vi "HOST_4651.vi"() -> ()   [LabVIEW 2018]
uses:
  <vilib>/userdefined/High Color/nirio_resource_hc.ctl
  <instrlib>/niDCPower/nidcpower.llb/niDCPower Measurement Type.ctl
  <vilib>/FPGAPlugInAG/PXI-7953R/niLvFpga_Open_PXI-7953R.vi
  <vilib>/rvi/interface/common/dynamic/niFpgaDynamicAddResources.vi
  <vilib>/FPGAPlugInAG/Dynamic/niLvFpga_Reset_Dynamic.vi
  <vilib>/FPGAPlugInAG/Dynamic/niLvFpga_Run_Dynamic.vi
  <vilib>/Utility/error.llb/Error Cluster From Error Code.vi
  <vilib>/rvi/errors/niLvFpgaAdjustHostInterfaceError.vi
  <vilib>/FPGAPlugInAG/Dynamic/niLvFpga_Close_Dynamic.vi
  <vilib>/rvi/interface/nirviOpenFPGA/nirviOpenFPGA.xnode
  FPGA Bitfiles/GMAX4651_FPGATarget_Target4651_7TB9TLSSPWg.lvbitx
  <vilib>/rvi/interface/nirviMethod/nirviMethod.xnode
  <vilib>/rvi/interface/nirviReadWriteControl/nirviReadWriteControl.xnode
  <vilib>/rvi/interface/nirviCloseFPGA/nirviCloseFPGA.xnode
  <vilib>/rvi/interface/Simulation/niFpgaSimulationCallBeginRW.vi
  NiFpgaLv.dll
  <vilib>/FPGAPlugInAG/Dynamic/niLvFpga_ReadFifo_Dynamic.vi
  <vilib>/rvi/errors/niLvFpgaMergeErrorWithErrorCode.vi
  <vilib>/FPGAPlugInAG/Dynamic/niLvFpga_StartFifo_Dynamic.vi
  <vilib>/FPGAPlugInAG/Dynamic/niLvFpga_WriteFifo_Dynamic.vi
panel:
  in  "Обнулить сбои":bool
  out "Прошили":bool
  out "НИ":bool
  out "FIFO_READ":i32
  out "Выкачали из памяти":bool
  in  "Проверка сбоев":bool
  out "SEU":u32
  in  "SPI":bool
  in  "Upd_WR":bool
  in  "W(T)/R(F)":bool
  out "READ":u8[](array[numeric])
  in  "Регистры":u8[](array[numeric])=[119, 12, 0, 1, 0, 0, 1, 0, 0, 0, 0, 0, 171, 23, 1, 0, 0, 4, 0, 24, 0, 120, 15, 0, 0, 0, 0, 0, 0, 0, 0, 0, 0, 0, 0, 0, 0, 0, 0, 0, 0, 0, 0, 0, 0, 0, 0, 0, 0, 0, 0, 0, 0, 0, 0, 0, 0, 0, 0, 0, 0, 0, 0, 0, 0, 0, 0, 0, 0, 0, 0, 0, 0, 0, 0, 0, 0, 0, 0, 0, 0, 0, 0, 172, 23, 0, 0, 6, 4, 4, 4, 196, 0, 32, 32, 4, 0, 5, 0, 5, 1, 4, 0, 139, 21, 255, 7, 1, 0, 0, 134, 1, 144, 2, 12, 0, 1, 236, 245, 255, 255, 114, 252, 255, 255, 255, 255, 255, 255, 255, 255, 255, 255, 255, 255, 255, 255, 255, 255, 255, 255, 118, 253, 255, 255, 255, 255, 255, 255, 255, 255, 249, 52, 244, 255, 255, 255, 255, 255, 255, 255, 255, 255, 255, 255, 255, 169, 252, 159, 202, 255, 217, 252, 159, 205, 255, 118, 253, 255, 255, 255, 118, 253, 255, 255, 255, 118, 253, 255, 255, 255, 118, 253, 255, 255, 255, 5, 196, 179, 79, 92, 5, 196, 179, 79, 92, 1, 12, 176, 192, 19, 105, 204, 245, 192, 20, 123, 220, 245, 196, 20, 115, 229, 213, 197, 255, 91, 124, 49, 192, 2, 87, 140, 241, 192, 19, 123, 220, 85, 68, 47, 5, 0, 241, 255, 255, 255, 255, 95, 192, 14, 5, 236, 0, 0, 0, 0, 0, 0, 0, 0, 0, 0, 0, 0, 0, 0, 0, 0, 0, 0, 0, 0, 0, 0, 0, 0, 0, 0, 0, 0, 0, 0, 0, 0, 0, 0, 0, 0, 0, 0, 0, 0, 0, 0, 0, 0, 0, 0, 0, 0, 0, 0, 0, 0, 0, 0, 0, 106, 1, 0, 0, 6, 27, 142, 9, 108, 57, 0, 0, 0, 0, 108, 57, 23, 15, 8, 1, 20, 0, 56, 71, 96, 68, 0, 0, 0, 0, 188, 194, 172, 160, 180, 148, 148, 200, 0, 160, 128, 148, 194, 66, 66, 64, 0, 0, 254, 254, 254, 254, 254, 254, 16, 160, 192, 0, 0, 0, 0, 0]
  in  "Адрес":u16
  in  "Кол-во":u16=370
  in  "Хватит ждать!":bool
  out "Записали адресов":u32
  out "Image":T1(plugin-control)
  out "世男":bool
  in  "FRAME!":bool
  in  "MOVIE":bool
  out "VGRSH":bool
  out "VDD33A":bool
  out "VGRSL":bool
  out "VDDCH":bool
  out "VTX1H":bool
  out "VDD33A":u16
  out "VDDCH":u16
  out "VTX1L":u16
  out "VDD13":u16
  in  "SEL_Time, ms":u32=100
  out "SEL":bool
  in  "VGRSH_selcur":dbl=0.07 caption="current limit" format="%_6p"
  in  "VDD33A_selcur":dbl=0.3 caption="current limit" format="%_6p"
  in  "VGRSL_selcur":dbl=0.03 caption="current limit" format="%_6p"
  in  "VDDCH_selcur":dbl=0.15 caption="current limit" format="%_6p"
  in  "VTX1H_selcur":dbl=0.2 caption="current limit" format="%_6p"
  in  "VTX1L_selcur":dbl=0.05 caption="current limit" format="%_6p"
  in  "VDDCL_RF_RS_selcur":dbl=0.1 caption="current limit" format="%_6p"
  in  "VDD13_selcur":dbl=0.99 caption="current limit" format="%_6p"
  in  "VDDPIX_selcur":dbl=0.5 caption="current limit" format="%_6p"
  out "VTX1L":bool
  out "VDDCL":bool
  out "VDD13":bool
  out "VDDPIX":bool
  in  "Период опроса, мс":u32=1
  in  "VDD33A, V":dbl=3.3 caption="voltage level" format="%_6p"
  in  "VDDCH, V":dbl=3.75 caption="voltage level" format="%_6p"
  in  "VTX1H, V":dbl=3.6 caption="voltage level" format="%_6p"
  in  "VDDCL_RF_RS, V":dbl=1.1 caption="voltage level" format="%_6p"
  in  "VDD33A_curlim":dbl=0.5 caption="current limit" format="%_6p"
  in  "VGRSL_curlim":dbl=0.1 caption="current limit" format="%_6p"
  in  "VDDCH_curlim":dbl=0.3 caption="current limit" format="%_6p"
  in  "VTX1H_curlim":dbl=0.3 caption="current limit" format="%_6p"
  in  "VTX1L_curlim":dbl=0.1 caption="current limit" format="%_6p"
  in  "VDDCL_RF_RS_curlim":dbl=0.2 caption="current limit" format="%_6p"
  in  "VGRSL, V":dbl=-1.0 caption="voltage level" format="%_6p"
  in  "VTX1L, V":dbl=-1.3 caption="voltage level" format="%_6p"
  out "VDD33A_char":dbl(graph)=2.9426590888639165e-06
  out "VGRSL_char":dbl(graph)=1.8968380980834295e-06
  out "VDDCH_char":dbl(graph)=0.00011100375072345994
  out "VTX1H_char":dbl(graph)=2.7759221072203326e-06
  out "VTX1L_char":dbl(graph)=-1.4343692569601055e-07
  out "VDDCL_RF_RS_char":dbl(graph)=7.705063078661294e-05
  in  "VDD13, V":dbl=1.3 caption="voltage level" format="%_6p"
  in  "VDD13_curlim":dbl=1.0 caption="current limit" format="%_6p"
  out "VDD13_char":dbl(graph)=-4.0587860431954116e-07
  in  "LED, V":dbl=-3.0 caption="voltage level" format="%_6p"
  in  "LED_curlim":dbl=0.05 caption="current limit" format="%_6p"
  out "LED_char":dbl(graph)=-1.6465603775405444e-06
  in  "VGRSH, V":dbl=4.1 caption="voltage level" format="%_6p"
  in  "VGRSH_curlim":dbl=0.1 caption="current limit" format="%_6p"
  out "VGRSH_char":dbl(graph)=7.96703589777135e-05
  in  "VDDPIX, V":dbl=3.9 caption="voltage level" format="%_6p"
  in  "VDDPIX_curlim":dbl=0.6 caption="current limit" format="%_6p"
  out "VDDPIX_char":dbl(graph)=4.6929457201886834e-05
  in  "3,3V_LVDS, V":dbl=3.3 caption="voltage level" format="%_6p"
  in  "3,3V_LVDS_curlim":dbl=0.1 caption="current limit" format="%_6p"
  out "3,3V_LVDS_char":dbl(graph)=1.0317150729546496e-06
  out "VGRSH_cur":dbl caption="measurement" format="%_6g"
  out "VDD33A_cur":dbl caption="measurement" format="%_6g"
  out "VGRSL_cur":dbl caption="measurement" format="%_6g"
  out "VDDCH_cur":dbl caption="measurement" format="%_6g"
  out "VTX1H_cur":dbl caption="measurement" format="%_6g"
  out "VTX1L_cur":dbl caption="measurement" format="%_6g"
  out "VDDCL_RF_RS_cur":dbl caption="measurement" format="%_6g"
  in  "LED":bool caption="output enabled"
  out "VDD13_cur":dbl caption="measurement" format="%_6g"
  out "VDDPIX_cur":dbl caption="measurement" format="%_6g"
  out "VGRSL":u16
  out "VDDPIX":u16
  out "VTX1H":u16
  out "VDDCL":u16
  out "VGRSH":u16
  in  "Стоп":bool
  in  "Питание":bool
  in  "SIM_SEL":bool
  in  "0":refnum<k15>="PXI1Slot2" caption="1"
  in  "1":refnum<k15>="PXI1Slot3"
  in  "2":refnum<k15>="PXI1Slot4" caption="1"
  in  "3":refnum<k15>="PXI1Slot5" caption="1"
  in  "resource name 2":T2="RIO0"
  in  "SEU":path=path "C:/LabView_PRJ/GMAX4651/SEU"
  in  "SEL":path=path "C:/LabView_PRJ/GMAX4651/SEL"
  out "Номер образца":string="0"
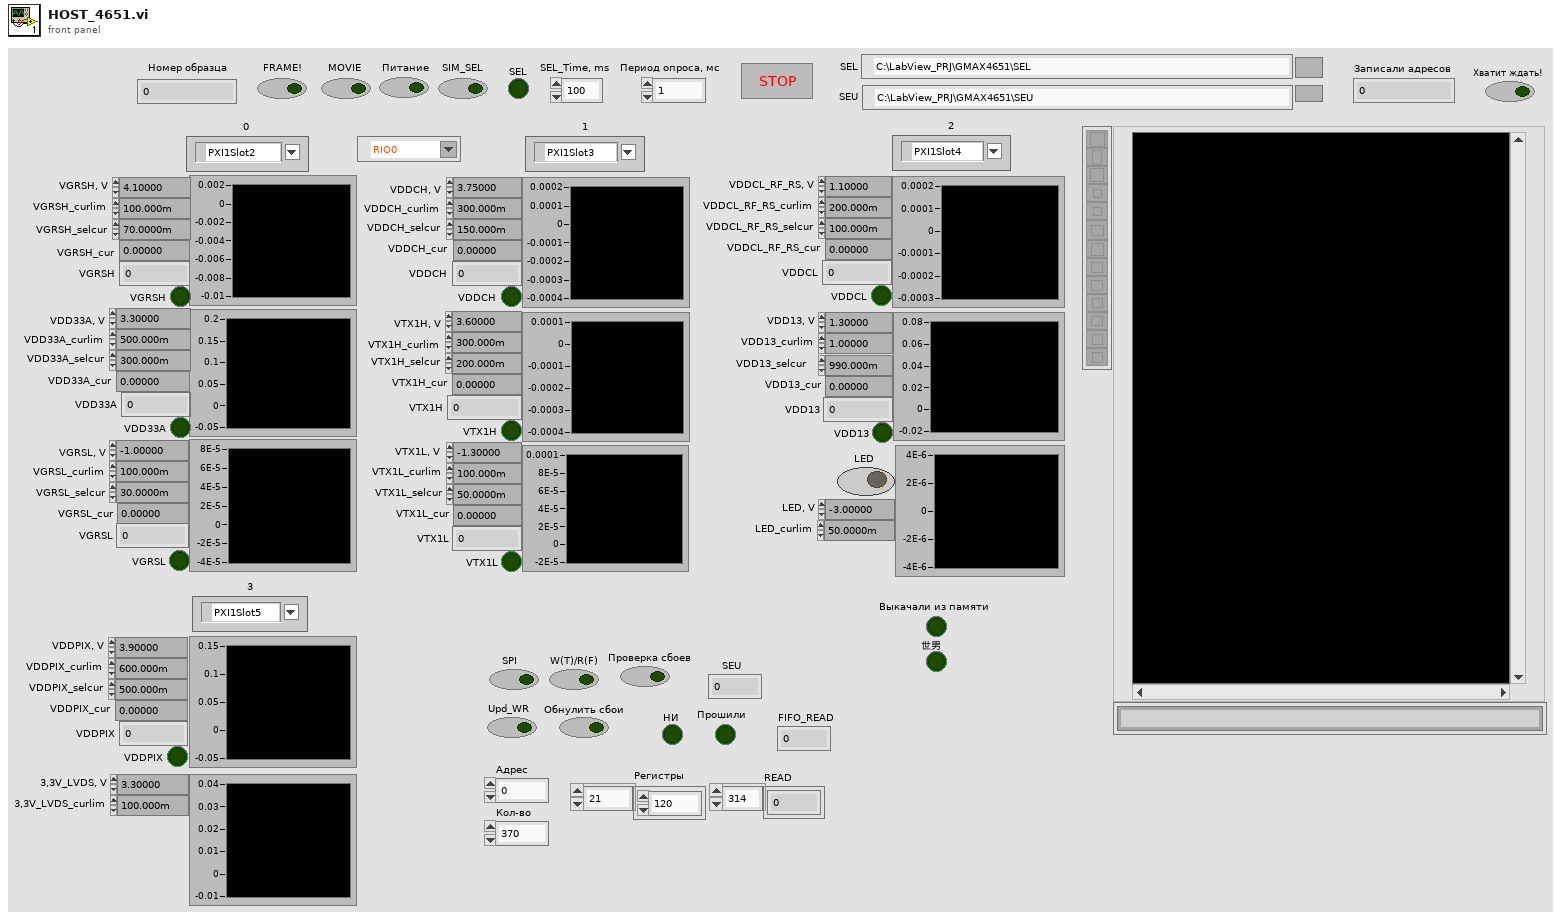
[diagram p1: front panel]
types:
  T1 = typedef "IMAQ Image.ctl" = refnum<image>
  T2 = typedef "nirio_resource_hc.ctl" = tag
  T3 = typedef "Image Type" = u32
  T4 = enum16{"open", "replace", "create", "open or create", "replace or create", "replace or create with confirmation"}
  T5 = typedef "niDCPower Measurement Type.ctl" = i32
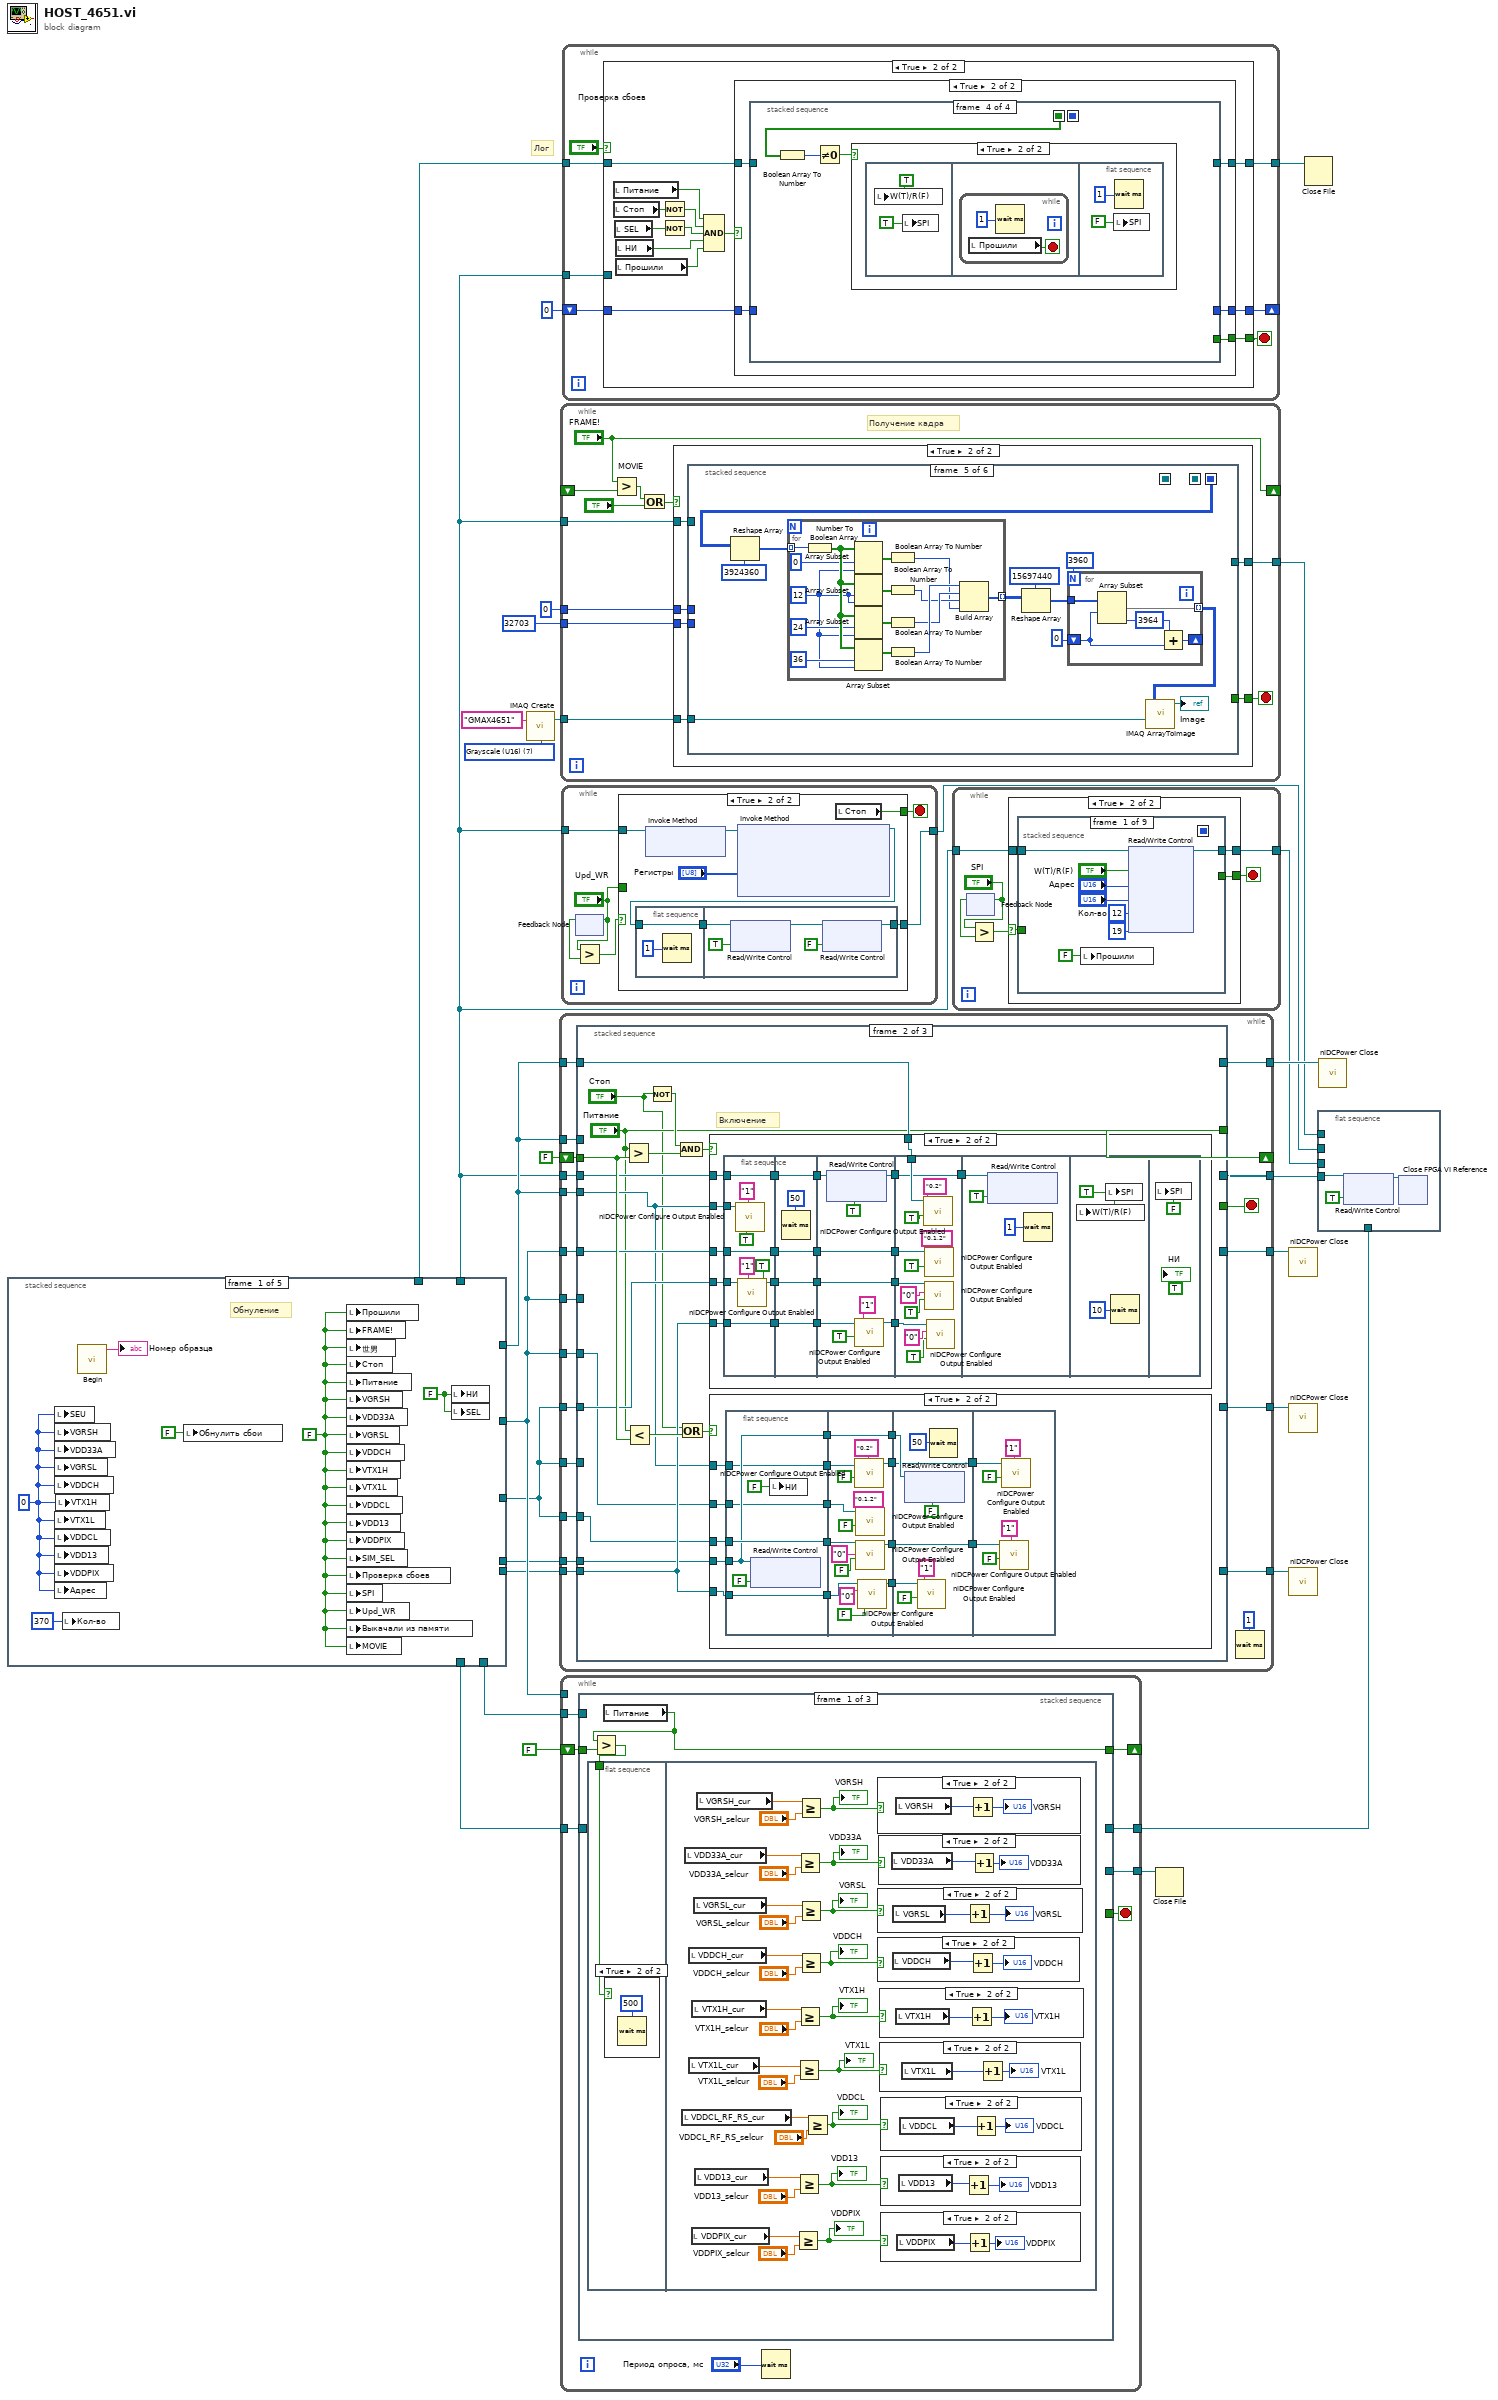
[diagram p0: block diagram]
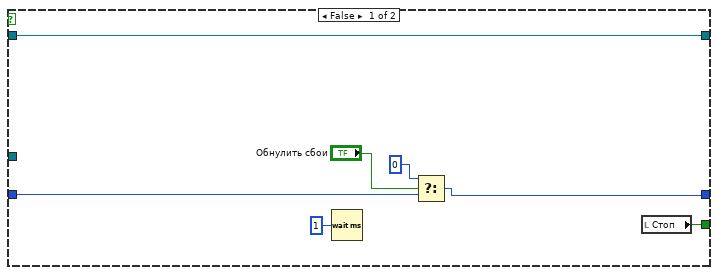
[diagram p2: hidden frame]
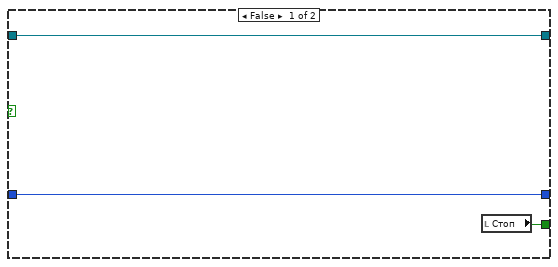
[diagram p3: hidden frame]
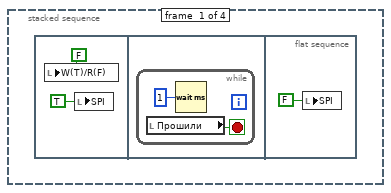
[diagram p4: hidden frame]
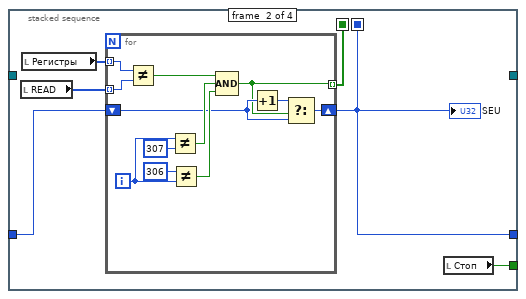
[diagram p5: hidden frame]
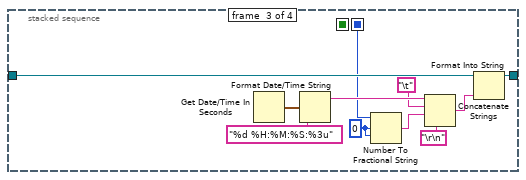
[diagram p6: hidden frame]
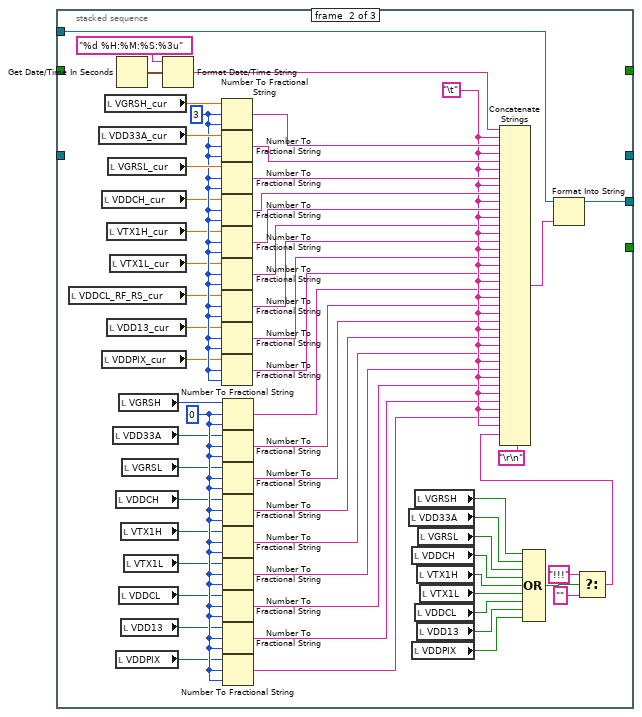
[diagram p18: hidden frame]
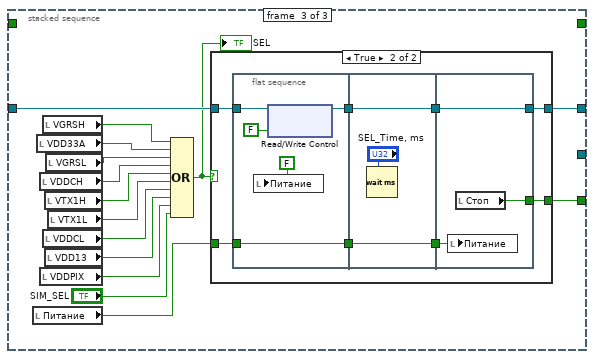
[diagram p19: hidden frame]
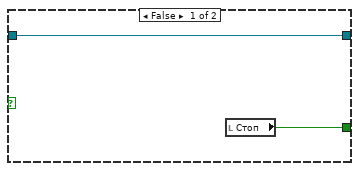
[diagram p20: hidden frame]
diagram:
  w13 = T3 7 items=["Grayscale (U8)", "Grayscale (I16)", "Grayscale (SGL)", "Complex (CSG)", "RGB (U32)", "HSL (U32)", "RGB (U64)", "Grayscale (U16)"] ("Image Type")
  # "Лог"
  n1 = stacked-sequence {
    tunnel: [_ _ _ _ w115] -> w19
    tunnel: [_ _ _ _ w108] -> w21
    tunnel: [_ _ _ _ w119] -> w20
    tunnel: [_ _ _ w103 _] -> w4
    tunnel: [_ _ _ w103 _] -> w16
    tunnel: [_ w42 _ _ _] -> w17
    tunnel: [_ _ _ _ w109] -> w18
    tunnel: [_ _ _ w103 _] -> w15
    tunnel: [_ _ w72 _ _] -> w3
    frame #0 {
      w31 = FALSE ("НИ")
      w30 = FALSE ("Стоп")
      w33 = u16 0 ("ADC")
      # "Обнуление"
      n2 = local write "SEU"(w33) -> ()
      n3 = local write "VGRSH"(w33) -> ()
      n4 = local write "VDD33A"(w33) -> ()
      n5 = local write "VGRSL"(w33) -> ()
      n6 = local write "VDDCH"(w33) -> ()
      n7 = local write "VTX1L"(w33) -> ()
      n8 = local write "VDDCL"(w33) -> ()
      n9 = local write "VDD13"(w33) -> ()
      n10 = local write "VDDPIX"(w33) -> ()
      n11 = local write "Адрес"(w33) -> ()
      n12 = local write "VTX1H"(w33) -> ()
      n13 = local write "Кол-во"(u16 370 ("Кол-во")) -> ()
      n14 = call "Begin.vi"() -> ("Номер образца 2"=→"Номер образца":string)  [unwired: 11 in]
      n15 = local write "Обнулить сбои"(FALSE ("Обнулить сбои")) -> ()
      n16 = local write "Прошили"(w30) -> ()
      n17 = local write "FRAME!"(w30) -> ()
      n18 = local write "世男"(w30) -> ()
      n19 = local write "Стоп"(w30) -> ()
      n20 = local write "Питание"(w30) -> ()
      n21 = local write "VGRSH"(w30) -> ()
      n22 = local write "VDD33A"(w30) -> ()
      n23 = local write "VGRSL"(w30) -> ()
      n24 = local write "VDDCH"(w30) -> ()
      n25 = local write "VTX1H"(w30) -> ()
      n26 = local write "VTX1L"(w30) -> ()
      n27 = local write "VDDCL"(w30) -> ()
      n28 = local write "VDD13"(w30) -> ()
      n29 = local write "VDDPIX"(w30) -> ()
      n30 = local write "SIM_SEL"(w30) -> ()
      n31 = local write "Проверка сбоев"(w30) -> ()
      n32 = local write "SPI"(w30) -> ()
      n33 = local write "Upd_WR"(w30) -> ()
      n34 = local write "Выкачали из памяти"(w30) -> ()
      n35 = local write "MOVIE"(w30) -> ()
      n36 = local write "НИ"(w31) -> ()
      n37 = local write "SEL"(w31) -> ()
    }
    frame #1 {
      w37 = "\t"
      # "Лог по токам"
      n38 = local read "Номер образца"() -> (w64:string)
      n39 = Build Path(base path="SEL", name or relative path=w64) -> (appended path=w61:path)
      n40 = Get Date/Time In Seconds() -> (seconds since 1Jan1904=w58:timestamp)
      n41 = call <vilib>:"Check if File or Folder Exists.vi"("path"=w61) -> ("file or folder exists?"=w62:bool, "dup path"=w63:path)  [unwired: 8 in, 1 out]
      n42 = Format Date/Time String(time format string (%c)="%d %H.%M.%S", seconds (now)=w58) -> (date/time string=w56:string)  [unwired: 1 in]
      n43 = case shown="False" w62 {
        tunnel: w63 -> [w70 w71]
        tunnel: [w69 w71] -> w36
        frame False {
          n44 = Create Folder(path (use dialog)=w70) -> (created path=w69:path)  [unwired: 2 in, 2 out]
        }
        frame True {
        }
      }
      n45 = Concatenate Strings(w56, ".xls" ("string")) -> (w55:string)
      n46 = Build Path(base path=w36, name or relative path=w55) -> (appended path=w57:path)
      n47 = Open/Create/Replace File(file path (use dialog)=w57, operation (0:open)=T4."open or create", access (0:read/write)=enum16{"read/write", "read-only", "write-only"}."read/write") -> (refnum out=w59:refnum<file>)  [unwired: 3 in, 2 out]
      n48 = case shown="True" TRUE {
        tunnel: w59 -> [w65 w68]
        tunnel: [w65 w66] -> w54
        frame False {
        }
        frame True {
          n49 = Set File Position(refnum=w68, from (0:start)=enum16{"start", "end", "current"}."end") -> (refnum out=w66:refnum<file>)  [unwired: 2 in, 1 out]
        }
      }
      n50 = Format Into String(initial string=w54, "Time" ("input 1"), w37, "VGRSH_cur", w37, "VDD33A_cur", w37, "VGRSL_cur", w37, "VDDCH_cur", w37, "VTX1H_cur", w37, "VTX1L_cur", w37, "VDDCL_RF_RS_cur", w37, "VDD13_cur", w37, "VDDPIX_cur", w37, "\r\n") -> (resulting string=w42:refnum<file>)  [unwired: 2 in, 1 out]
    }
    frame #2 {
      w75 = "\t"
      # "Лог по сбоям"
      n51 = local read "Номер образца"() -> (w79:string)
      n52 = Build Path(base path="SEU", name or relative path=w79) -> (appended path=w93:path)
      n53 = Get Date/Time In Seconds() -> (seconds since 1Jan1904=w91:timestamp)
      n54 = call <vilib>:"Check if File or Folder Exists.vi"("path"=w93) -> ("file or folder exists?"=w94:bool, "dup path"=w95:path)  [unwired: 8 in, 1 out]
      n55 = Format Date/Time String(time format string (%c)="%d %H.%M.%S", seconds (now)=w91) -> (date/time string=w89:string)  [unwired: 1 in]
      n56 = case shown="False" w94 {
        tunnel: w95 -> [w101 w102]
        tunnel: [w100 w102] -> w80
        frame False {
          n57 = Create Folder(path (use dialog)=w101) -> (created path=w100:path)  [unwired: 2 in, 2 out]
        }
        frame True {
        }
      }
      n58 = Concatenate Strings(w89, ".xls" ("string")) -> (w88:string)
      n59 = Build Path(base path=w80, name or relative path=w88) -> (appended path=w90:path)
      n60 = Open/Create/Replace File(file path (use dialog)=w90, operation (0:open)=T4."open or create", access (0:read/write)=enum16{"read/write", "read-only", "write-only"}."read/write") -> (refnum out=w92:refnum<file>)  [unwired: 3 in, 2 out]
      n61 = case shown="True" TRUE {
        tunnel: w92 -> [w96 w99]
        tunnel: [w96 w97] -> w87
        frame False {
        }
        frame True {
          n62 = Set File Position(refnum=w99, from (0:start)=enum16{"start", "end", "current"}."end") -> (refnum out=w97:refnum<file>)  [unwired: 2 in, 1 out]
        }
      }
      n63 = Format Into String(initial string=w87, "Time" ("input 1"), w75, "Регистр №" ("input 3"), w75, "Содержание" ("input 4"), w75, "Кол-во сбоев" ("input 7"), "\r\n") -> (resulting string=w72:refnum<file>)  [unwired: 2 in, 1 out]
    }
    frame #3 {
      n64 = xnode "Open FPGA VI Reference"("resource name"="resource name 2") -> ("FPGA VI Reference Out"=w104:refnum<k20>)  [unwired: 1 in, 1 out]
      n65 = xnode "Invoke Method"("FPGA VI Reference In"=w104) -> ("FPGA VI Reference Out"=w107:refnum<k20>, "error out"=w106:errorcluster)  [unwired: 1 in]
      n66 = xnode "Invoke Method"("FPGA VI Reference In"=w107, "error in"=w106) -> ("FPGA VI Reference Out"=w103:refnum<k20>)  [unwired: 1 in, 1 out]
    }
    frame #4 {
      n67 = call <instrlib>:"niDCPower Initialize.vi"("resource name"="2") -> ("error out"=w125:errorcluster, "instrument handle out"=w122:refnum<k15>)  [unwired: 3 in, 6 out]
      n68 = call <instrlib>:"niDCPower Initialize.vi"("resource name"="1") -> ("error out"=w123:errorcluster, "instrument handle out"=w120:refnum<k15>)  [unwired: 3 in, 6 out]
      n69 = call <instrlib>:"niDCPower Initialize.vi"("resource name"="3") -> ("error out"=w113:errorcluster, "instrument handle out"=w114:refnum<k15>)  [unwired: 3 in, 6 out]
      n70 = call <instrlib>:"niDCPower Initialize.vi"("resource name"="0") -> ("error out"=w124:errorcluster, "instrument handle out"=w121:refnum<k15>)  [unwired: 3 in, 6 out]
      n71 = call <instrlib>:"niDCPower Configure Voltage Level.vi"("error in (no error)"=w125, "voltage level"=0.0, "channel name"="0,1,2", "instrument handle"=w122) -> ("instrument handle out"=w115:refnum<k15>)  [unwired: 6 in, 1 out]
      n72 = call <instrlib>:"niDCPower Configure Voltage Level.vi"("error in (no error)"=w123, "voltage level"=0.0, "channel name"="0,1,2", "instrument handle"=w120) -> ("instrument handle out"=w119:refnum<k15>)  [unwired: 6 in, 1 out]
      n73 = call <instrlib>:"niDCPower Configure Voltage Level.vi"("error in (no error)"=w113, "voltage level"=0.0, "channel name"="0,1", "instrument handle"=w114) -> ("instrument handle out"=w109:refnum<k15>)  [unwired: 6 in, 1 out]
      n74 = call <instrlib>:"niDCPower Configure Voltage Level.vi"("error in (no error)"=w124, "voltage level"=0.0, "channel name"="0,1,2", "instrument handle"=w121) -> ("instrument handle out"=w108:refnum<k15>)  [unwired: 6 in, 1 out]
    }
  }
  n75 = call "IMAQ Create"("Image Name"="GMAX4651", "Image Type"=w13) -> ("New Image"=w10:T1)  [unwired: 3 in, 1 out]
  n76 = while {
    shift-right: [w151] -> _
    shift-left: FALSE -> [w152]
    tunnel: w21 -> [w150]
    tunnel: w20 -> [w144]
    tunnel: w19 -> [w141]
    tunnel: w18 -> [w149]
    tunnel: w21 -> [w146]
    tunnel: w21 -> [w145]
    tunnel: w20 -> [w143]
    tunnel: w20 -> [w142]
    tunnel: w19 -> [w140]
    tunnel: w19 -> [w139]
    tunnel: [w138] -> w25
    tunnel: [w137] -> w26
    tunnel: [w136] -> w27
    tunnel: [w135] -> w28
    tunnel: w4 -> [w134]
    tunnel: w15 -> [w133]
    tunnel: [w132] -> w5
    stop <- w148 stop-if-true
    n77 = stacked-sequence {
      tunnel: w152 -> [_ w271 _]
      tunnel: [_ "Питание" _] -> w151
      tunnel: w150 -> [w164 w258 w392]
      tunnel: w149 -> [w153 w263 w389]
      tunnel: [_ _ w393] -> w148
      tunnel: w146 -> [w163 _ _]
      tunnel: w145 -> [w162 w260 _]
      tunnel: w144 -> [w161 w266 w391]
      tunnel: w143 -> [w160 _ _]
      tunnel: w142 -> [w159 w261 _]
      tunnel: w141 -> [w158 w265 w390]
      tunnel: w140 -> [w157 _ _]
      tunnel: w139 -> [w156 w262 _]
      tunnel: [_ _ w392] -> w138
      tunnel: [_ _ w391] -> w137
      tunnel: [_ _ w390] -> w136
      tunnel: [_ _ w389] -> w135
      tunnel: w134 -> [_ w259 w388]
      tunnel: w133 -> [_ w257 _]
      tunnel: [_ _ w388] -> w132
      frame #0 {
        w178 = T5 0 items=["Current", "Voltage"] ("measurement type")
        n78 = call <instrlib>:"niDCPower Configure Current Limit.vi"("current limit"="VGRSH_curlim", "channel name"="0", "instrument handle"=w164) -> ("instrument handle out"=w195:refnum<k15>)  [unwired: 7 in, 1 out]
        n79 = call <instrlib>:"niDCPower Configure Current Limit.vi"("current limit"="VDD33A_curlim", "channel name"="1", "instrument handle"=w163) -> ("instrument handle out"=w235:refnum<k15>)  [unwired: 7 in, 1 out]
        n80 = call <instrlib>:"niDCPower Configure Current Limit.vi"("current limit"="VGRSL_curlim", "channel name"="2", "instrument handle"=w162) -> ("instrument handle out"=w236:refnum<k15>)  [unwired: 7 in, 1 out]
        n81 = call <instrlib>:"niDCPower Configure Current Limit.vi"("current limit"="VDDCH_curlim", "channel name"="0", "instrument handle"=w161) -> ("instrument handle out"=w237:refnum<k15>)  [unwired: 7 in, 1 out]
        n82 = call <instrlib>:"niDCPower Configure Current Limit.vi"("current limit"="VTX1H_curlim", "channel name"="1", "instrument handle"=w160) -> ("instrument handle out"=w238:refnum<k15>)  [unwired: 7 in, 1 out]
        n83 = call <instrlib>:"niDCPower Configure Current Limit.vi"("current limit"="VTX1L_curlim", "channel name"="2", "instrument handle"=w159) -> ("instrument handle out"=w239:refnum<k15>)  [unwired: 7 in, 1 out]
        n84 = call <instrlib>:"niDCPower Configure Current Limit.vi"("current limit"="VDDCL_RF_RS_curlim", "channel name"="0", "instrument handle"=w158) -> ("instrument handle out"=w240:refnum<k15>)  [unwired: 7 in, 1 out]
        n85 = call <instrlib>:"niDCPower Configure Current Limit.vi"("current limit"="VDD13_curlim", "channel name"="1", "instrument handle"=w157) -> ("instrument handle out"=w208:refnum<k15>)  [unwired: 7 in, 1 out]
        n86 = call <instrlib>:"niDCPower Configure Current Limit.vi"("current limit"="LED_curlim", "channel name"="2", "instrument handle"=w156) -> ("instrument handle out"=w203:refnum<k15>)  [unwired: 7 in, 1 out]
        n87 = call <instrlib>:"niDCPower Configure Current Limit.vi"("current limit"="VDDPIX_curlim", "channel name"="0", "instrument handle"=w153) -> ("instrument handle out"=w188:refnum<k15>)  [unwired: 7 in, 1 out]
        n88 = call <instrlib>:"niDCPower Configure Current Limit.vi"("current limit"="3,3V_LVDS_curlim", "channel name"="1", "instrument handle"=w153) -> ("instrument handle out"=w183:refnum<k15>)  [unwired: 7 in, 1 out]
        n89 = call <instrlib>:"niDCPower Configure Voltage Level.vi"("voltage level"="VGRSH, V", "channel name"="0", "instrument handle"=w195) -> ("instrument handle out"=w198:refnum<k15>)  [unwired: 7 in, 1 out]
        n90 = call <instrlib>:"niDCPower Configure Voltage Level.vi"("voltage level"="VDD33A, V", "channel name"="1", "instrument handle"=w235) -> ("instrument handle out"=w218:refnum<k15>)  [unwired: 7 in, 1 out]
        n91 = call <instrlib>:"niDCPower Configure Voltage Level.vi"("voltage level"="VGRSL, V", "channel name"="2", "instrument handle"=w236) -> ("instrument handle out"=w217:refnum<k15>)  [unwired: 7 in, 1 out]
        n92 = call <instrlib>:"niDCPower Configure Voltage Level.vi"("voltage level"="VDDCH, V", "channel name"="0", "instrument handle"=w237) -> ("instrument handle out"=w216:refnum<k15>)  [unwired: 7 in, 1 out]
        n93 = call <instrlib>:"niDCPower Configure Voltage Level.vi"("voltage level"="VTX1H, V", "channel name"="1", "instrument handle"=w238) -> ("instrument handle out"=w215:refnum<k15>)  [unwired: 7 in, 1 out]
        n94 = call <instrlib>:"niDCPower Configure Voltage Level.vi"("voltage level"="VTX1L, V", "channel name"="2", "instrument handle"=w239) -> ("instrument handle out"=w214:refnum<k15>)  [unwired: 7 in, 1 out]
        n95 = call <instrlib>:"niDCPower Configure Voltage Level.vi"("voltage level"="VDDCL_RF_RS, V", "channel name"="0", "instrument handle"=w240) -> ("instrument handle out"=w213:refnum<k15>)  [unwired: 7 in, 1 out]
        n96 = call <instrlib>:"niDCPower Configure Voltage Level.vi"("voltage level"="VDD13, V", "channel name"="1", "instrument handle"=w208) -> ("instrument handle out"=w211:refnum<k15>)  [unwired: 7 in, 1 out]
        n97 = call <instrlib>:"niDCPower Configure Voltage Level.vi"("voltage level"="LED, V", "channel name"="2", "instrument handle"=w203) -> ("instrument handle out"=w200:refnum<k15>)  [unwired: 7 in, 1 out]
        n98 = call <instrlib>:"niDCPower Configure Voltage Level.vi"("voltage level"="VDDPIX, V", "channel name"="0", "instrument handle"=w188) -> ("instrument handle out"=w191:refnum<k15>)  [unwired: 7 in, 1 out]
        n99 = call <instrlib>:"niDCPower Configure Voltage Level.vi"("voltage level"="3,3V_LVDS, V", "channel name"="1", "instrument handle"=w183) -> ("instrument handle out"=w180:refnum<k15>)  [unwired: 7 in, 1 out]
        n100 = call <instrlib>:"niDCPower Measure.vi"("measurement type"=w178, "channel name"="0", "instrument handle"=w198) -> ("measurement"=→"VGRSH_char" →"VGRSH_cur":dbl)  [unwired: 6 in, 2 out]
        n101 = call <instrlib>:"niDCPower Measure.vi"("measurement type"=w178, "channel name"="1", "instrument handle"=w218) -> ("measurement"=→"VDD33A_char" →"VDD33A_cur":dbl)  [unwired: 6 in, 2 out]
        n102 = call <instrlib>:"niDCPower Measure.vi"("measurement type"=w178, "channel name"="2", "instrument handle"=w217) -> ("measurement"=→"VGRSL_char" →"VGRSL_cur":dbl)  [unwired: 6 in, 2 out]
        n103 = call <instrlib>:"niDCPower Measure.vi"("measurement type"=w178, "channel name"="0", "instrument handle"=w216) -> ("measurement"=→"VDDCH_char" →"VDDCH_cur":dbl)  [unwired: 6 in, 2 out]
        n104 = call <instrlib>:"niDCPower Measure.vi"("measurement type"=w178, "channel name"="1", "instrument handle"=w215) -> ("measurement"=→"VTX1H_char" →"VTX1H_cur":dbl)  [unwired: 6 in, 2 out]
        n105 = call <instrlib>:"niDCPower Measure.vi"("measurement type"=w178, "channel name"="2", "instrument handle"=w214) -> ("measurement"=→"VTX1L_char" →"VTX1L_cur":dbl)  [unwired: 6 in, 2 out]
        n106 = call <instrlib>:"niDCPower Measure.vi"("measurement type"=w178, "channel name"="0", "instrument handle"=w213) -> ("measurement"=→"VDDCL_RF_RS_char" →"VDDCL_RF_RS_cur":dbl)  [unwired: 6 in, 2 out]
        n107 = call <instrlib>:"niDCPower Measure.vi"("measurement type"=w178, "channel name"="1", "instrument handle"=w211) -> ("measurement"=→"VDD13_char" →"VDD13_cur":dbl)  [unwired: 6 in, 2 out]
        n108 = call <instrlib>:"niDCPower Measure.vi"("measurement type"=w178, "channel name"="2", "instrument handle"=w200) -> ("measurement"=→"LED_char":dbl, "instrument handle out"=w166:refnum<k15>)  [unwired: 6 in, 1 out]
        n109 = call <instrlib>:"niDCPower Measure.vi"("measurement type"=w178, "channel name"="0", "instrument handle"=w191) -> ("measurement"=→"VDDPIX_char" →"VDDPIX_cur":dbl)  [unwired: 6 in, 2 out]
        n110 = call <instrlib>:"niDCPower Measure.vi"("measurement type"=w178, "channel name"="1", "instrument handle"=w180) -> ("measurement"=→"3,3V_LVDS_char":dbl)  [unwired: 6 in, 2 out]
        n111 = call <instrlib>:"niDCPower Configure Output Enabled.vi"("output enabled"="LED", "channel name"="2", "instrument handle"=w166) -> ()  [unwired: 7 in, 2 out]
      }
      frame #1 {
        # "Включение"
        n112 = Greater?(x="Питание", y=w271) -> (0:w269:bool)
        n113 = Less?(x="Питание", y=w271) -> (x < y?=w267:bool)
        n114 = Not(x="Стоп") -> (.not. x?=w268:bool)
        n115 = And(x=w268, y=w269) -> (x .and. y?=w270:bool)
        n116 = Or(x="Стоп", y=w267) -> (x .or. y?=w264:bool)
        n117 = case shown="True" w270 {
          tunnel: w266 -> [_ w336]
          tunnel: w265 -> [_ w342]
          tunnel: w260 -> [_ w343]
          tunnel: w263 -> [_ w330]
          tunnel: w259 -> [_ w341]
          tunnel: w258 -> [_ w338]
          frame False {
          }
          frame True {
            n118 = flat-sequence {
              tunnel: w343 -> [w353]
              tunnel: w342 -> [w350]
              tunnel: w341 -> [w347]
              tunnel: [w347] -> w339
              tunnel: [w346] -> w337
              tunnel: w336 -> [w346]
              tunnel: [w345] -> w331
              tunnel: w330 -> [w344]
              tunnel: [w344] -> w329
              tunnel: [w357] -> w340
              tunnel: w339 -> [w357]
              tunnel: w337 -> [w356]
              tunnel: [w356] -> w335
              tunnel: [w355] -> w332
              tunnel: w331 -> [w355]
              tunnel: w329 -> [w354]
              tunnel: [w354] -> w328
              tunnel: w340 -> [w367]
              tunnel: w335 -> [w365]
              tunnel: [w365] -> w334
              tunnel: [w364] -> w333
              tunnel: w332 -> [w364]
              tunnel: w328 -> [w362]
              tunnel: [w361] -> w327
              tunnel: [w363] -> w325
              tunnel: w338 -> [w379]
              tunnel: w334 -> [w377]
              tunnel: w333 -> [w372]
              tunnel: w327 -> [w370]
              tunnel: [w368] -> w326
              tunnel: w325 -> [w368]
              tunnel: w326 -> [w383]
              frame #0 {
                n119 = call <instrlib>:"niDCPower Configure Output Enabled.vi"("output enabled"=TRUE, "channel name"="1", "instrument handle"=w353) -> ()  [unwired: 7 in, 2 out]
                n120 = call <instrlib>:"niDCPower Configure Output Enabled.vi"("output enabled"=TRUE, "channel name"="1", "instrument handle"=w350) -> ("instrument handle out"=w345:refnum<k15>)  [unwired: 7 in, 1 out]
              }
              frame #1 {
                n121 = Wait (ms)(milliseconds to wait=u32 50) -> ()  [unwired: 1 out]
              }
              frame #2 {
                n122 = xnode "Read/Write Control"("FPGA VI Reference In"=w367, "Автомат"=TRUE) -> ("FPGA VI Reference Out"=w363:refnum<k20>)  [unwired: 1 in, 1 out]
                n123 = call <instrlib>:"niDCPower Configure Output Enabled.vi"("output enabled"=TRUE, "channel name"="1", "instrument handle"=w362) -> ("instrument handle out"=w361:refnum<k15>)  [unwired: 7 in, 1 out]
              }
              frame #3 {
                n124 = call <instrlib>:"niDCPower Configure Output Enabled.vi"("output enabled"=TRUE, "channel name"="0,2", "instrument handle"=w379) -> ()  [unwired: 7 in, 2 out]
                n125 = call <instrlib>:"niDCPower Configure Output Enabled.vi"("output enabled"=TRUE, "channel name"="0,1,2", "instrument handle"=w377) -> ()  [unwired: 7 in, 2 out]
                n126 = call <instrlib>:"niDCPower Configure Output Enabled.vi"("output enabled"=TRUE, "channel name"="0", "instrument handle"=w372) -> ()  [unwired: 7 in, 2 out]
                n127 = call <instrlib>:"niDCPower Configure Output Enabled.vi"("output enabled"=TRUE, "channel name"="0", "instrument handle"=w370) -> ()  [unwired: 7 in, 2 out]
              }
              frame #4 {
                n128 = xnode "Read/Write Control"("FPGA VI Reference In"=w383, "SYS_RST_N"=TRUE) -> ()  [unwired: 1 in, 2 out]
                n129 = Wait (ms)(milliseconds to wait=u32 1) -> ()  [unwired: 1 out]
              }
              frame #5 {
                w384 = TRUE ("SPI")
                n130 = local write "W(T)/R(F)"(w384) -> ()
                n131 = local write "SPI"(w384) -> ()
                n132 = Wait (ms)(milliseconds to wait=u32 10) -> ()  [unwired: 1 out]
              }
              frame #6 {
                n133 = local write "SPI"(FALSE ("SPI")) -> ()
                "НИ" <- TRUE ("НИ")
              }
            }
          }
        }
        n134 = case shown="True" w264 {
          tunnel: w261 -> [_ w277]
          tunnel: w262 -> [_ w283]
          tunnel: w260 -> [_ w279]
          tunnel: w263 -> [_ w285]
          tunnel: w257 -> [_ w287]
          frame False {
          }
          frame True {
            n135 = flat-sequence {
              tunnel: w287 -> [w291]
              tunnel: [w293] -> w286
              tunnel: w285 -> [w293]
              tunnel: [w292] -> w284
              tunnel: w283 -> [w292]
              tunnel: [w291] -> w281
              tunnel: [w290] -> w280
              tunnel: w279 -> [w290]
              tunnel: [w289] -> w278
              tunnel: w277 -> [w289]
              tunnel: w286 -> [w304]
              tunnel: w284 -> [w303]
              tunnel: [w302] -> w282
              tunnel: w281 -> [w302]
              tunnel: w280 -> [w301]
              tunnel: w278 -> [w300]
              tunnel: [w297] -> w275
              tunnel: [w296] -> w273
              tunnel: [w295] -> w272
              tunnel: w282 -> [w317]
              tunnel: [w315] -> w276
              tunnel: w275 -> [w315]
              tunnel: [w314] -> w274
              tunnel: w273 -> [w314]
              tunnel: w272 -> [w313]
              tunnel: w276 -> [w322]
              tunnel: w274 -> [w321]
              frame #0 {
                n136 = xnode "Read/Write Control"("FPGA VI Reference In"=w291, "SYS_RST_N"=FALSE) -> ()  [unwired: 1 in, 2 out]
                n137 = local write "НИ"(FALSE ("НИ")) -> ()
              }
              frame #1 {
                n138 = call <instrlib>:"niDCPower Configure Output Enabled.vi"("output enabled"=FALSE, "channel name"="0,2", "instrument handle"=w301) -> ("instrument handle out"=w297:refnum<k15>)  [unwired: 7 in, 1 out]
                n139 = call <instrlib>:"niDCPower Configure Output Enabled.vi"("output enabled"=FALSE, "channel name"="0,1,2", "instrument handle"=w300) -> ()  [unwired: 7 in, 2 out]
                n140 = call <instrlib>:"niDCPower Configure Output Enabled.vi"("output enabled"=FALSE, "channel name"="0", "instrument handle"=w303) -> ("instrument handle out"=w296:refnum<k15>)  [unwired: 7 in, 1 out]
                n141 = call <instrlib>:"niDCPower Configure Output Enabled.vi"("output enabled"=FALSE, "channel name"="0", "instrument handle"=w304) -> ("instrument handle out"=w295:refnum<k15>)  [unwired: 7 in, 1 out]
              }
              frame #2 {
                n142 = xnode "Read/Write Control"("FPGA VI Reference In"=w317, "Автомат"=FALSE) -> ()  [unwired: 1 in, 2 out]
                n143 = call <instrlib>:"niDCPower Configure Output Enabled.vi"("output enabled"=FALSE, "channel name"="1", "instrument handle"=w313) -> ()  [unwired: 7 in, 2 out]
                n144 = Wait (ms)(milliseconds to wait=u32 50) -> ()  [unwired: 1 out]
              }
              frame #3 {
                n145 = call <instrlib>:"niDCPower Configure Output Enabled.vi"("output enabled"=FALSE, "channel name"="1", "instrument handle"=w321) -> ()  [unwired: 7 in, 2 out]
                n146 = call <instrlib>:"niDCPower Configure Output Enabled.vi"("output enabled"=FALSE, "channel name"="1", "instrument handle"=w322) -> ()  [unwired: 7 in, 2 out]
              }
            }
          }
        }
      }
      frame #2 {
        n147 = local read "Стоп"() -> (w393:bool)
      }
    }
    n148 = Wait (ms)(milliseconds to wait=u32 1) -> ()  [unwired: 1 out]
  }
  n149 = while {
    tunnel: w4 -> [w395]
    shift-right: ["FRAME!"] -> _
    shift-left: _ -> [w404]
    tunnel: u32 0 -> [w401]
    tunnel: u32 32703 ("163840") -> [w400]
    tunnel: w10 -> [w397]
    tunnel: [w394] -> w6
    stop <- w396 stop-if-true
    # "Получение кадра"
    n150 = Greater?(x="FRAME!", y=w404) -> (0:w403:bool)
    n151 = Or(x=w403, y="MOVIE") -> (x .or. y?=w402:bool)
    n152 = case shown="True" w402 {
      tunnel: w401 -> [_ w413]
      tunnel: w400 -> [_ w412]
      tunnel: w397 -> [_ w411]
      tunnel: [w406 w410] -> w396
      tunnel: w395 -> [w405 w409]
      tunnel: [w405 w408] -> w394
      frame False {
        n153 = Wait (ms)(milliseconds to wait=u32 1) -> ()  [unwired: 1 out]
        n154 = local read "Стоп"() -> (w406:bool)
      }
      frame True {
        n155 = stacked-sequence {
          seq-local: [w416 _ _ _ _ _] -> [_ w434 _ _ _ _]
          seq-local: [_ w433 _ _ _ _] -> [_ _ w446 _ _ _]
          seq-local: [_ _ w444 _ _ _] -> [_ _ _ _ w500 _]
          tunnel: w413 -> [_ _ w447 _ _ _]
          tunnel: w412 -> [_ _ w445 _ _ _]
          tunnel: w411 -> [_ _ _ _ w492 _]
          tunnel: [_ _ _ _ _ w523] -> w410
          tunnel: w409 -> [w414 _ _ _ _ _]
          tunnel: [_ _ w443 _ _ _] -> w408
          frame #0 {
            # "Почистили FIFO"
            n156 = xnode "Invoke Method"("FPGA VI Reference In"=w414, "Number of Elements"=u32 0, "Timeout (ms)"=0) -> ("FPGA VI Reference Out"=w418:refnum<k20>, "Elements Remaining"=w419:u32)  [unwired: 1 in, 2 out]
            n157 = xnode "Invoke Method"("FPGA VI Reference In"=w418, "Number of Elements"=w419, "Timeout (ms)"=0) -> ("FPGA VI Reference Out"=w417:refnum<k20>)  [unwired: 1 in, 3 out]
            n158 = flat-sequence {
              tunnel: w417 -> [w428]
              tunnel: [w424] -> w415
              tunnel: [w430] -> w416
              tunnel: w415 -> [w429]
              frame #0 {
                n159 = xnode "Read/Write Control"("FPGA VI Reference In"=w428, "Кадр в память"=TRUE ("EXPOSURE")) -> ("FPGA VI Reference Out"=w424:refnum<k20>)  [unwired: 1 in, 1 out]
                n160 = Wait (ms)(milliseconds to wait=u32 1) -> ()  [unwired: 1 out]
                "世男" <- FALSE
                "Выкачали из памяти" <- FALSE ("Выкачали из памяти")
              }
              frame #1 {
                n161 = xnode "Read/Write Control"("FPGA VI Reference In"=w429, "Кадр в память"=FALSE) -> ("FPGA VI Reference Out"=w430:refnum<k20>)  [unwired: 1 in, 1 out]
                n162 = Wait (ms)(milliseconds to wait=u32 1) -> ()  [unwired: 1 out]
              }
            }
          }
          frame #1 {
            n163 = while {
              tunnel: [w441] -> w433
              tunnel: w434 -> [w440]
              stop <- w437 stop-if-true
              n164 = xnode "Read/Write Control"("FPGA VI Reference In"=w440) -> ("FPGA VI Reference Out"=w441:refnum<k20>, "Записали адресов"=w436:u32)  [unwired: 1 in, 1 out]
              "Записали адресов" <- w436
              n165 = Wait (ms)(milliseconds to wait=u32 1) -> ()  [unwired: 1 out]
              n166 = Greater?(x=w436, y=u32 3924000) -> (0:w438:bool)
              n167 = Or(x=w438, y="Хватит ждать!") -> (x .or. y?=w437:bool)
            }
          }
          frame #2 {
            n168 = for {
              N: 120 -> [_]
              tunnel: w446 -> [w456]
              shift-right: [w453] -> _
              shift-left: w447 -> [w455]
              shift-right: [w452] -> _
              shift-left: w445 -> [w454]
              tunnel: [w451] -> w444 mode=indexing
              tunnel: [w450] -> w443
              tunnel: w445 -> [w449]
              n169 = stacked-sequence {
                seq-local: [w458 _ _ _ _] -> [_ w465 _ _ _]
                seq-local: [_ w464 _ _ _] -> [_ _ w468 _ _]
                seq-local: [_ _ w467 _ _] -> [_ _ _ w472 _]
                seq-local: [_ _ _ w471 _] -> [_ _ _ _ w483]
                tunnel: w456 -> [w463 _ _ _ _]
                tunnel: w455 -> [w462 _ _ _ _]
                tunnel: w454 -> [w461 _ _ _ _]
                tunnel: [w460 _ _ _ _] -> w453
                tunnel: [w459 _ _ _ _] -> w452
                tunnel: [_ _ _ _ w485] -> w451
                tunnel: [_ _ _ _ w484] -> w450
                tunnel: w449 -> [w457 _ _ _ _]
                frame #0 {
                  n170 = xnode "Read/Write Control"("FPGA VI Reference In"=w463, "Нач_адр"=w462, "Кон_адр"=w461) -> ("FPGA VI Reference Out"=w458:refnum<k20>)  [unwired: 1 in, 1 out]
                  n171 = Add(x=w462, y=w457) -> (x+y=w460:u32)
                  n172 = Add(x=w457, y=w461) -> (x+y=w459:u32)
                }
                frame #1 {
                  n173 = xnode "Read/Write Control"("FPGA VI Reference In"=w465, "Кадр на ПК"=TRUE ("HOST")) -> ("FPGA VI Reference Out"=w464:refnum<k20>)  [unwired: 1 in, 1 out]
                }
                frame #2 {
                  n174 = xnode "Read/Write Control"("FPGA VI Reference In"=w468, "Кадр на ПК"=FALSE ("HOST")) -> ("FPGA VI Reference Out"=w467:refnum<k20>)  [unwired: 1 in, 1 out]
                }
                frame #3 {
                  n175 = Get Date/Time In Seconds() -> (seconds since 1Jan1904=w470:timestamp)
                  n176 = while {
                    tunnel: w472 -> [w481]
                    tunnel: [w480] -> w471
                    tunnel: w470 -> [w478]
                    stop <- w473 stop-if-true
                    # "Записан FIFO?"
                    n177 = Get Date/Time In Seconds() -> (seconds since 1Jan1904=w479:timestamp)
                    n178 = xnode "Read/Write Control"("FPGA VI Reference In"=w481) -> ("FPGA VI Reference Out"=w480:refnum<k20>, "Записали FIFO"=w475:bool)  [unwired: 1 in, 1 out]
                    n179 = Subtract(x=w479, y=w478) -> (x-y=w477:dbl)
                    n180 = Greater?(x=w477, y=5.0) -> (0:w474:bool)
                    n181 = Or(x=w475, y=w474) -> (x .or. y?=w473:bool)
                    n182 = Wait (ms)(milliseconds to wait=u32 1) -> ()  [unwired: 1 out]
                  }
                }
                frame #4 {
                  n183 = xnode "Invoke Method"("FPGA VI Reference In"=w483, "Number of Elements"=u32 0, "Timeout (ms)"=0) -> ("FPGA VI Reference Out"=w489:refnum<k20>, "Elements Remaining"=w490:u32)  [unwired: 1 in, 2 out]
                  n184 = xnode "Invoke Method"("FPGA VI Reference In"=w489, "Number of Elements"=w490, "Timeout (ms)"=0) -> ("FPGA VI Reference Out"=w484:refnum<k20>, "Data"=w485:u64[])  [unwired: 1 in, 2 out]
                }
              }
            }
          }
          frame #3 {
            n185 = local write "Выкачали из памяти"(TRUE ("Выкачали из памяти")) -> ()
          }
          frame #4 {
            n186 = Reshape Array(w500, 3924360 ("dimension size")) -> (w502:u64[])
            n187 = for {
              tunnel: w502 -> [w522] mode=indexing
              tunnel: [w516] -> w499 mode=indexing
              w517 = 12 ("index")
              n188 = Number To Boolean Array(number=w522) -> (Boolean array=w521:bool[])
              n189 = Array Subset(array=w521, index=0, length=w517) -> (w511:bool[])
              n190 = Array Subset(array=w521, index=w517, length=w517) -> (w510:bool[])
              n191 = Array Subset(array=w521, index=24, length=w517) -> (w509:bool[])
              n192 = Array Subset(array=w521, index=36, length=w517) -> (w508:bool[])
              n193 = Boolean Array To Number(Boolean array=w511) -> (number=w512:u16)
              n194 = Boolean Array To Number(Boolean array=w510) -> (number=w513:u16)
              n195 = Boolean Array To Number(Boolean array=w509) -> (number=w514:u16)
              n196 = Boolean Array To Number(Boolean array=w508) -> (number=w515:u16)
              n197 = Build Array(w515, w514, w513, w512) -> (w516:u16[])
            }
            n198 = Reshape Array(w499, 15697440 ("dimension size")) -> (w493:u16[])
            n199 = for {
              N: 3960 ("6032") -> [_]
              shift-right: [w507] -> _
              shift-left: 0 ("index") -> [w506]
              tunnel: [w505] -> w497 mode=indexing
              tunnel: w493 -> [w503]
              w504 = 3964 ("3964")
              n200 = Array Subset(array=w503, index=w506, length=w504) -> (w505:u16[])
              n201 = Add(x=w504, y=w506) -> (x+y=w507:i32)
            }
            n202 = call "IMAQ ArrayToImage"("Image Pixels (U16)"=w497, "Image"=w492) -> ("Image Out"=→"Image":T1)  [unwired: 8 in, 1 out]
          }
          frame #5 {
            n203 = local write "世男"(TRUE ("世男")) -> ()
            n204 = local read "Стоп"() -> (w523:bool)
          }
        }
      }
    }
  }
  n205 = while {
    tunnel: w16 -> [w527]
    shift-right: [w531] -> _
    shift-left: FALSE ("Питание") -> [w532]
    tunnel: w17 -> [w529]
    tunnel: [w526] -> w23
    tunnel: [w525] -> w9
    tunnel: w20 -> [_]
    stop <- w528 stop-if-true
    n206 = stacked-sequence {
      tunnel: w532 -> [w535 _ _]
      tunnel: [w534 _ _] -> w531
      tunnel: w529 -> [_ w636 _]
      tunnel: [_ _ w656] -> w528
      tunnel: w527 -> [_ _ w655]
      tunnel: [_ w625 _] -> w526
      tunnel: [_ _ w653] -> w525
      frame #0 {
        n207 = flat-sequence {
          tunnel: w533 -> [w536]
          frame #0 {
            n208 = case shown="True" w536 {
              frame False {
              }
              frame True {
                n209 = Wait (ms)(milliseconds to wait=u32 500) -> ()  [unwired: 1 out]
              }
            }
          }
          frame #1 {
            n210 = local read "VDDCL_RF_RS_cur"() -> (w549:dbl)
            n211 = local read "VDD33A_cur"() -> (w558:dbl)
            n212 = local read "VDDCH_cur"() -> (w560:dbl)
            n213 = local read "VTX1L_cur"() -> (w550:dbl)
            n214 = local read "VDDPIX_cur"() -> (w547:dbl)
            n215 = local read "VTX1H_cur"() -> (w551:dbl)
            n216 = local read "VGRSL_cur"() -> (w559:dbl)
            n217 = local read "VDD13_cur"() -> (w548:dbl)
            n218 = local read "VGRSH_cur"() -> (w557:dbl)
            n219 = Greater Or Equal?(x=w547, y="VDDPIX_selcur") -> (x >= y?=w543:bool)
            "VDDPIX" <- w543
            n220 = Greater Or Equal?(x=w550, y="VTX1L_selcur") -> (x >= y?=w546:bool)
            "VTX1L" <- w546
            n221 = Greater Or Equal?(x=w548, y="VDD13_selcur") -> (x >= y?=w544:bool)
            "VDD13" <- w544
            n222 = Greater Or Equal?(x=w558, y="VDD33A_selcur") -> (x >= y?=w541:bool)
            "VDD33A" <- w541
            n223 = Greater Or Equal?(x=w551, y="VTX1H_selcur") -> (x >= y?=w538:bool)
            "VTX1H" <- w538
            n224 = Greater Or Equal?(x=w557, y="VGRSH_selcur") -> (x >= y?=w542:bool)
            "VGRSH" <- w542
            n225 = Greater Or Equal?(x=w559, y="VGRSL_selcur") -> (x >= y?=w540:bool)
            "VGRSL" <- w540
            n226 = Greater Or Equal?(x=w560, y="VDDCH_selcur") -> (x >= y?=w539:bool)
            "VDDCH" <- w539
            n227 = Greater Or Equal?(x=w549, y="VDDCL_RF_RS_selcur") -> (x >= y?=w545:bool)
            "VDDCL" <- w545
            n228 = case shown="True" w542 {
              frame False {
              }
              frame True {
                n229 = local read "VGRSH"() -> (w581:u16)
                n230 = Increment(x=w581) -> (x+1=→"VGRSH":u16)
              }
            }
            n231 = case shown="True" w540 {
              frame False {
              }
              frame True {
                n232 = local read "VGRSL"() -> (w577:u16)
                n233 = Increment(x=w577) -> (x+1=→"VGRSL":u16)
              }
            }
            n234 = case shown="True" w539 {
              frame False {
              }
              frame True {
                n235 = local read "VDDCH"() -> (w576:u16)
                n236 = Increment(x=w576) -> (x+1=→"VDDCH":u16)
              }
            }
            n237 = case shown="True" w541 {
              frame False {
              }
              frame True {
                n238 = local read "VDD33A"() -> (w580:u16)
                n239 = Increment(x=w580) -> (x+1=→"VDD33A":u16)
              }
            }
            n240 = case shown="True" w538 {
              frame False {
              }
              frame True {
                n241 = local read "VTX1H"() -> (w574:u16)
                n242 = Increment(x=w574) -> (x+1=→"VTX1H":u16)
              }
            }
            n243 = case shown="True" w546 {
              frame False {
              }
              frame True {
                n244 = local read "VTX1L"() -> (w572:u16)
                n245 = Increment(x=w572) -> (x+1=→"VTX1L":u16)
              }
            }
            n246 = case shown="True" w545 {
              frame False {
              }
              frame True {
                n247 = local read "VDDCL"() -> (w570:u16)
                n248 = Increment(x=w570) -> (x+1=→"VDDCL":u16)
              }
            }
            n249 = case shown="True" w544 {
              frame False {
              }
              frame True {
                n250 = local read "VDD13"() -> (w567:u16)
                n251 = Increment(x=w567) -> (x+1=→"VDD13":u16)
              }
            }
            n252 = case shown="True" w543 {
              frame False {
              }
              frame True {
                n253 = local read "VDDPIX"() -> (w566:u16)
                n254 = Increment(x=w566) -> (x+1=→"VDDPIX":u16)
              }
            }
          }
        }
        n255 = local read "Питание"() -> (w534:bool)
        n256 = Greater?(x=w534, y=w535) -> (0:w533:bool)
      }
      frame #1 {
        w611 = "\t"
        w623 = i16 0 ("width (-)")
        w624 = i16 3 ("width (-)")
        n257 = local read "VDDCL_RF_RS_cur"() -> (w619:dbl)
        n258 = local read "VDD33A_cur"() -> (w634:dbl)
        n259 = local read "VDDCH_cur"() -> (w622:dbl)
        n260 = local read "VDDPIX_cur"() -> (w617:dbl)
        n261 = local read "VGRSH_cur"() -> (w635:dbl)
        n262 = local read "VTX1H_cur"() -> (w621:dbl)
        n263 = local read "VDD13_cur"() -> (w618:dbl)
        n264 = local read "VGRSL_cur"() -> (w626:dbl)
        n265 = local read "VTX1L_cur"() -> (w620:dbl)
        n266 = local read "VDD33A"() -> (w615:u16)
        n267 = local read "VDDCH"() -> (w613:u16)
        n268 = local read "VDDPIX"() -> (w588:u16)
        n269 = Get Date/Time In Seconds() -> (seconds since 1Jan1904=w641:timestamp)
        n270 = local read "VGRSH"() -> (w616:u16)
        n271 = local read "VDDCL"() -> (w590:u16)
        n272 = local read "VTX1H"() -> (w612:u16)
        n273 = local read "VDD13"() -> (w589:u16)
        n274 = local read "VGRSL"() -> (w614:u16)
        n275 = local read "VTX1L"() -> (w591:u16)
        n276 = Format Date/Time String(time format string (%c)="%d %H:%M:%S:%3u", seconds (now)=w641) -> (date/time string=w633:string)  [unwired: 1 in]
        n277 = Number To Fractional String(number=w635, width (-)=w624, precision (6)=w624) -> (F-format string=w632:string)  [unwired: 1 in]
        n278 = Number To Fractional String(number=w634, width (-)=w624, precision (6)=w624) -> (F-format string=w631:string)  [unwired: 1 in]
        n279 = Number To Fractional String(number=w626, width (-)=w624, precision (6)=w624) -> (F-format string=w630:string)  [unwired: 1 in]
        n280 = Number To Fractional String(number=w622, width (-)=w624, precision (6)=w624) -> (F-format string=w629:string)  [unwired: 1 in]
        n281 = Number To Fractional String(number=w621, width (-)=w624, precision (6)=w624) -> (F-format string=w628:string)  [unwired: 1 in]
        n282 = Number To Fractional String(number=w620, width (-)=w624, precision (6)=w624) -> (F-format string=w610:string)  [unwired: 1 in]
        n283 = Number To Fractional String(number=w619, width (-)=w624, precision (6)=w624) -> (F-format string=w609:string)  [unwired: 1 in]
        n284 = Number To Fractional String(number=w618, width (-)=w624, precision (6)=w624) -> (F-format string=w608:string)  [unwired: 1 in]
        n285 = Number To Fractional String(number=w617, width (-)=w624, precision (6)=w624) -> (F-format string=w607:string)  [unwired: 1 in]
        n286 = Number To Fractional String(number=w616, width (-)=w623, precision (6)=w623) -> (F-format string=w606:string)  [unwired: 1 in]
        n287 = Number To Fractional String(number=w615, width (-)=w623, precision (6)=w623) -> (F-format string=w605:string)  [unwired: 1 in]
        n288 = Number To Fractional String(number=w614, width (-)=w623, precision (6)=w623) -> (F-format string=w604:string)  [unwired: 1 in]
        n289 = Number To Fractional String(number=w613, width (-)=w623, precision (6)=w623) -> (F-format string=w603:string)  [unwired: 1 in]
        n290 = Number To Fractional String(number=w612, width (-)=w623, precision (6)=w623) -> (F-format string=w602:string)  [unwired: 1 in]
        n291 = Number To Fractional String(number=w591, width (-)=w623, precision (6)=w623) -> (F-format string=w601:string)  [unwired: 1 in]
        n292 = Number To Fractional String(number=w590, width (-)=w623, precision (6)=w623) -> (F-format string=w600:string)  [unwired: 1 in]
        n293 = Number To Fractional String(number=w589, width (-)=w623, precision (6)=w623) -> (F-format string=w599:string)  [unwired: 1 in]
        n294 = Number To Fractional String(number=w588, width (-)=w623, precision (6)=w623) -> (F-format string=w598:string)  [unwired: 1 in]
        n295 = local read "VDD33A"() -> (w584:bool)
        n296 = local read "VDDCH"() -> (w586:bool)
        n297 = local read "VDDPIX"() -> (w592:bool)
        n298 = local read "VGRSH"() -> (w583:bool)
        n299 = local read "VDDCL"() -> (w594:bool)
        n300 = local read "VTX1H"() -> (w587:bool)
        n301 = local read "VDD13"() -> (w593:bool)
        n302 = local read "VGRSL"() -> (w585:bool)
        n303 = local read "VTX1L"() -> (w595:bool)
        n304 = Compound Arithmetic op=OR(w583, w584, w585, w586, w587, w595, w594, w593, w592) -> (w627:bool)
        n305 = Select(t="!!!", s=w627, f="") -> (s? t:f=w597:string)
        n306 = Concatenate Strings(w633, w611, w632, w611, w631, w611, w630, w611, w629, w611, w628, w611, w610, w611, w609, w611, w608, w611, w607, w611, w606, w611, w605, w611, w604, w611, w603, w611, w602, w611, w601, w611, w600, w611, w599, w611, w598, w611, w597, "\r\n") -> (w637:string)
        n307 = Format Into String(initial string=w636, w637) -> (resulting string=w625:refnum<file>)  [unwired: 2 in, 1 out]
      }
      frame #2 {
        n308 = local read "Питание"() -> (w654:bool)
        n309 = local read "VDD33A"() -> (w650:bool)
        n310 = local read "VDDCH"() -> (w648:bool)
        n311 = local read "VDDPIX"() -> (w643:bool)
        n312 = local read "VGRSH"() -> (w651:bool)
        n313 = local read "VDDCL"() -> (w645:bool)
        n314 = local read "VTX1H"() -> (w647:bool)
        n315 = local read "VDD13"() -> (w644:bool)
        n316 = local read "VGRSL"() -> (w649:bool)
        n317 = local read "VTX1L"() -> (w646:bool)
        n318 = Compound Arithmetic op=OR(w651, w650, w649, w648, w647, w646, w645, w644, w643, "SIM_SEL") -> (w652:bool)
        "SEL" <- w652
        n319 = case shown="True" w652 {
          tunnel: [w658 w666] -> w656
          tunnel: w655 -> [w657 w665]
          tunnel: w654 -> [_ w662]
          tunnel: [w657 w661] -> w653
          frame False {
            n320 = local read "Стоп"() -> (w658:bool)
          }
          frame True {
            n321 = flat-sequence {
              tunnel: w665 -> [w670]
              tunnel: [w668] -> w663
              tunnel: w662 -> [w668]
              tunnel: [w667] -> w659
              tunnel: [w673] -> w664
              tunnel: w663 -> [w673]
              tunnel: [w672] -> w660
              tunnel: w659 -> [w672]
              tunnel: [w677] -> w666
              tunnel: w664 -> [w676]
              tunnel: [w675] -> w661
              tunnel: w660 -> [w675]
              frame #0 {
                n322 = local write "Питание"(FALSE ("Питание")) -> ()
                n323 = xnode "Read/Write Control"("FPGA VI Reference In"=w670, "Автомат"=FALSE ("Линейки")) -> ("FPGA VI Reference Out"=w667:refnum<k20>)  [unwired: 1 in, 1 out]
              }
              frame #1 {
                n324 = Wait (ms)(milliseconds to wait="SEL_Time, ms") -> ()  [unwired: 1 out]
              }
              frame #2 {
                n325 = local write "Питание"(w676) -> ()
                n326 = local read "Стоп"() -> (w677:bool)
              }
            }
          }
        }
      }
    }
    n327 = Wait (ms)(milliseconds to wait="Период опроса, мс") -> ()  [unwired: 1 out]
  }
  n328 = while {
    tunnel: w4 -> [w680]
    tunnel: [w678] -> w7
    stop <- w682 stop-if-true
    n329 = feedback-in #1("Upd_WR") -> ()
    n330 = feedback #1() -> (w683:bool)  [unwired: 1 in]
    n331 = Greater?(x="Upd_WR", y=w683) -> (0:w681:bool)
    n332 = case shown="True" w681 {
      tunnel: [w685 w692] -> w682
      tunnel: w680 -> [w684 w689]
      tunnel: "Upd_WR" -> [_ _]
      tunnel: [w684 w687] -> w678
      frame False {
        n333 = Wait (ms)(milliseconds to wait=u32 50) -> ()  [unwired: 1 out]
        n334 = local read "Стоп"() -> (w685:bool)
      }
      frame True {
        n335 = flat-sequence {
          tunnel: w691 -> [w695]
          tunnel: [w695] -> w688
          tunnel: w688 -> [w700]
          tunnel: [w696] -> w687
          frame #0 {
            n336 = Wait (ms)(milliseconds to wait=u32 1) -> ()  [unwired: 1 out]
          }
          frame #1 {
            n337 = xnode "Read/Write Control"("FPGA VI Reference In"=w700, "Upd_WR"=TRUE) -> ("FPGA VI Reference Out"=w699:refnum<k20>)  [unwired: 1 in, 1 out]
            n338 = xnode "Read/Write Control"("FPGA VI Reference In"=w699, "Upd_WR"=FALSE) -> ("FPGA VI Reference Out"=w696:refnum<k20>)  [unwired: 1 in, 1 out]
          }
        }
        n339 = xnode "Invoke Method"("FPGA VI Reference In"=w689) -> ("FPGA VI Reference Out"=w690:refnum<k20>)  [unwired: 1 in, 1 out]
        n340 = xnode "Invoke Method"("FPGA VI Reference In"=w690, "Data"="Регистры") -> ("FPGA VI Reference Out"=w691:refnum<k20>)  [unwired: 2 in, 2 out]
        n341 = local read "Стоп"() -> (w692:bool)
      }
    }
  }
  n342 = while {
    tunnel: w4 -> [w707]
    tunnel: w3 -> [w706]
    tunnel: [w705] -> w2
    shift-right: [w701] -> _
    shift-left: u32 0 -> [w702]
    stop <- w703 stop-if-true
    n343 = case shown="True" "Проверка сбоев" {
      tunnel: [w712 w719] -> w703
      tunnel: w707 -> [_ _]
      tunnel: w706 -> [w713 w720]
      tunnel: [w713 w716] -> w705
      tunnel: w702 -> [w710 w718]
      tunnel: [w709 w717] -> w701
      frame False {
        n344 = Wait (ms)(milliseconds to wait=u32 1) -> ()  [unwired: 1 out]
        n345 = Select(t=u32 0, s="Обнулить сбои", f=w710) -> (s? t:f=w709:u32)
        n346 = local read "Стоп"() -> (w712:bool)
      }
      frame True {
        n347 = local read "Питание"() -> (w725:bool)
        n348 = local read "Стоп"() -> (w727:bool)
        n349 = local read "SEL"() -> (w726:bool)
        n350 = local read "НИ"() -> (w722:bool)
        n351 = local read "Прошили"() -> (w715:bool)
        n352 = Not(x=w727) -> (.not. x?=w724:bool)
        n353 = Not(x=w726) -> (.not. x?=w723:bool)
        n354 = Compound Arithmetic op=AND(w725, w724, w723, w722, w715) -> (w721:bool)
        n355 = case shown="True" w721 {
          tunnel: w720 -> [w728 w735]
          tunnel: [w730 w734] -> w719
          tunnel: w718 -> [w729 w733]
          tunnel: [w729 w732] -> w717
          tunnel: [w728 w731] -> w716
          frame False {
            n356 = local read "Стоп"() -> (w730:bool)
          }
          frame True {
            n357 = stacked-sequence {
              seq-local: [_ w742 _ _] -> [_ _ w763 _]
              seq-local: [_ w741 _ _] -> [_ _ _ w772]
              tunnel: w735 -> [_ _ w768 _]
              tunnel: [_ w746 _ _] -> w734
              tunnel: w733 -> [_ w743 _ _]
              tunnel: [_ w742 _ _] -> w732
              tunnel: [_ _ w759 _] -> w731
              frame #0 {
                n358 = flat-sequence {
                  frame #0 {
                    n359 = local write "W(T)/R(F)"(FALSE) -> ()
                    n360 = local write "SPI"(TRUE ("SPI")) -> ()
                  }
                  frame #1 {
                    n361 = while {
                      stop <- w739 stop-if-true
                      n362 = local read "Прошили"() -> (w739:bool)
                      n363 = Wait (ms)(milliseconds to wait=u32 1) -> ()  [unwired: 1 out]
                    }
                  }
                  frame #2 {
                    n364 = local write "SPI"(FALSE ("SPI")) -> ()
                  }
                }
              }
              frame #1 {
                n365 = local read "READ"() -> (w745:u8[])
                n366 = local read "Регистры"() -> (w744:u8[])
                n367 = for {
                  tunnel: w745 -> [w751] mode=indexing
                  tunnel: w744 -> [w758] mode=indexing
                  shift-right: [w748] -> w742
                  shift-left: w743 -> [w749]
                  tunnel: [w747] -> w741 mode=indexing
                  i -> [w752]
                  n368 = Not Equal?(x=w758, y=w751) -> (x != y?=w755:bool)
                  n369 = Not Equal?(x=w752, y=307) -> (x != y?=w754:bool)
                  n370 = Not Equal?(x=306, y=w752) -> (x != y?=w753:bool)
                  n371 = Compound Arithmetic op=AND(w755, w754, w753) -> (w747:bool)
                  n372 = Increment(x=w749) -> (x+1=w750:u32)
                  n373 = Select(t=w750, s=w747, f=w749) -> (s? t:f=w748:u32)
                }
                "SEU" <- w742
                n374 = local read "Стоп"() -> (w746:bool)
              }
              frame #2 {
                w762 = i16 0 ("width (-)")
                n375 = Get Date/Time In Seconds() -> (seconds since 1Jan1904=w767:timestamp)
                n376 = Format Date/Time String(time format string (%c)="%d %H:%M:%S:%3u", seconds (now)=w767) -> (date/time string=w765:string)  [unwired: 1 in]
                n377 = Number To Fractional String(number=w763, width (-)=w762, precision (6)=w762) -> (F-format string=w761:string)  [unwired: 1 in]
                n378 = Concatenate Strings(w765, "\t", w761, "\r\n") -> (w769:string)
                n379 = Format Into String(initial string=w768, w769) -> (resulting string=w759:refnum<file>)  [unwired: 2 in, 1 out]
              }
              frame #3 {
                n380 = Boolean Array To Number(Boolean array=w772) -> (number=w771:u32)
                n381 = Not Equal To 0?(x=w771) -> (x != 0?=w770:bool)
                n382 = case shown="True" w770 {
                  frame False {
                  }
                  frame True {
                    n383 = flat-sequence {
                      frame #0 {
                        n384 = local write "W(T)/R(F)"(TRUE) -> ()
                        n385 = local write "SPI"(TRUE ("SPI")) -> ()
                      }
                      frame #1 {
                        n386 = while {
                          stop <- w776 stop-if-true
                          n387 = local read "Прошили"() -> (w776:bool)
                          n388 = Wait (ms)(milliseconds to wait=u32 1) -> ()  [unwired: 1 out]
                        }
                      }
                      frame #2 {
                        n389 = local write "SPI"(FALSE ("SPI")) -> ()
                        n390 = Wait (ms)(milliseconds to wait=u32 1) -> ()  [unwired: 1 out]
                      }
                    }
                  }
                }
              }
            }
          }
        }
      }
    }
  }
  n391 = while {
    tunnel: w4 -> [w781]
    tunnel: [w779] -> w8
    stop <- w780 stop-if-true
    n392 = feedback #2() -> (w784:bool)  [unwired: 1 in]
    n393 = feedback-in #2("SPI") -> ()
    n394 = Greater?(x="SPI", y=w784) -> (0:w782:bool)
    n395 = case shown="True" w782 {
      selector: w782 -> [_ w790]
      tunnel: w781 -> [w785 w791]
      tunnel: [w787 w789] -> w780
      tunnel: [w785 w788] -> w779
      frame False {
        n396 = Wait (ms)(milliseconds to wait=u32 1) -> ()  [unwired: 1 out]
        n397 = local read "Стоп"() -> (w787:bool)
      }
      frame True {
        n398 = stacked-sequence {
          seq-local: [_ _ _ _ _ _ _ w810 _] -> [_ _ _ _ _ _ _ _ w817]
          tunnel: w791 -> [w799 _ w802 _ w806 _ w809 w813 w818]
          tunnel: w790 -> [_ _ _ _ _ _ _ _ _]
          tunnel: [_ _ _ _ _ _ _ _ w819] -> w789
          tunnel: [w793 _ _ _ _ _ _ _ _] -> w788
          frame #0 {
            n399 = local write "Прошили"(FALSE ("Прошили")) -> ()
            n400 = xnode "Read/Write Control"("FPGA VI Reference In"=w799, "W(T)/R(F)"="W(T)/R(F)", "Адрес"="Адрес", "Кол-во"="Кол-во", "12"=u8 12, "FR"=u8 19) -> ("FPGA VI Reference Out"=w793:refnum<k20>)  [unwired: 1 in, 1 out]
          }
          frame #1 {
            n401 = Wait (ms)(milliseconds to wait=u32 1) -> ()  [unwired: 1 out]
          }
          frame #2 {
            n402 = xnode "Read/Write Control"("FPGA VI Reference In"=w802, "SPI"=TRUE) -> ()  [unwired: 1 in, 2 out]
          }
          frame #3 {
            n403 = Wait (ms)(milliseconds to wait=u32 1) -> ()  [unwired: 1 out]
          }
          frame #4 {
            n404 = xnode "Read/Write Control"("FPGA VI Reference In"=w806, "SPI"=FALSE, "Upd_RD"=TRUE) -> ()  [unwired: 1 in, 2 out]
          }
          frame #5 {
            n405 = Wait (ms)(milliseconds to wait=u32 1) -> ()  [unwired: 1 out]
          }
          frame #6 {
            n406 = xnode "Read/Write Control"("FPGA VI Reference In"=w809, "Upd_RD"=FALSE) -> ()  [unwired: 1 in, 2 out]
          }
          frame #7 {
            n407 = xnode "Invoke Method"("FPGA VI Reference In"=w813, "Number of Elements"=u32 0, "Timeout (ms)"=0) -> ("Elements Remaining"=w810:u32)  [unwired: 1 in, 3 out]
            "FIFO_READ" <- w810
          }
          frame #8 {
            n408 = xnode "Invoke Method"("FPGA VI Reference In"=w818, "Number of Elements"=w817, "Timeout (ms)"=0) -> ("Data"=→"READ":u8[])  [unwired: 1 in, 3 out]
            n409 = local read "Стоп"() -> (w819:bool)
            "Прошили" <- TRUE ("Прошили")
          }
        }
      }
    }
  }
  n410 = Close File(refnum=w23) -> ()  [unwired: 1 in, 2 out]
  n411 = call <instrlib>:"niDCPower Close.vi"("instrument handle"=w26) -> ()  [unwired: 10 in, 1 out]
  n412 = call <instrlib>:"niDCPower Close.vi"("instrument handle"=w27) -> ()  [unwired: 10 in, 1 out]
  n413 = call <instrlib>:"niDCPower Close.vi"("instrument handle"=w28) -> ()  [unwired: 10 in, 1 out]
  n414 = Close File(refnum=w2) -> ()  [unwired: 1 in, 2 out]
  n415 = flat-sequence {
    tunnel: w9 -> [_]
    tunnel: w8 -> [_]
    tunnel: w7 -> [_]
    tunnel: w6 -> [_]
    tunnel: w5 -> [w820]
    frame #0 {
      n416 = xnode "Read/Write Control"("FPGA VI Reference In"=w820, "Стоп"=TRUE) -> ("FPGA VI Reference Out"=w822:refnum<k20>)  [unwired: 1 in, 1 out]
      n417 = xnode "Close FPGA VI Reference"("FPGA VI Reference In"=w822) -> ()  [unwired: 1 in, 1 out]
    }
  }
  n418 = call <instrlib>:"niDCPower Close.vi"("instrument handle"=w25) -> ()  [unwired: 10 in, 1 out]
